vi "Begin.vi"(8 "error in":errorcluster) -> (0 "error out":errorcluster)   [LabVIEW 2016]
doc: "Called before other user functions, this VI is expected to open initial I/O refnums, load in file data, and do all program initialization. Notice that the <B>error out</B> terminal is simply used for data flow. Wiring it to other structures or subVIs ensures that this VI runs first."
uses:
  <vilib>/Rock Robotics/WPI/DriverStation/WPI_DriverStationRobotMode2.ctl
  <vilib>/Rock Robotics/WPI/Joystick/WPI_JoystickDeviceEnum.ctl
  <vilib>/Rock Robotics/SystemInterfaces/spilib/spi_bus.ctl
  <vilib>/Rock Robotics/WPI/SafetyOutput/WPI_SafetyOutputConfigMenu.ctl
  <vilib>/Rock Robotics/SystemInterfaces/DIO/FPGA_DIOPWMChannel.ctl
  <vilib>/Rock Robotics/WPI/Solenoid/WPI_SolenoidChannel.ctl
  <vilib>/Rock Robotics/SystemInterfaces/DIO/FPGA_DIOChannel.ctl
  <vilib>/Rock Robotics/WPI/Encoder/WPI_EncoderType.ctl
  <vilib>/Rock Robotics/SystemInterfaces/AI/FPGA_AIChannel.ctl
  Robot Global Data.vi
  navX Library v2/IO/Open/Z900_navX_Open_SPI.vi
  <vilib>/Rock Robotics/WPI/MotorControl/WPI_MotorControlOpen VictorSP.vi
  <vilib>/Rock Robotics/WPI/Solenoid/WPI_SolenoidOpenSingle.vi
  <vilib>/Rock Robotics/WPI/RobotDrive/WPI_RobotDriveOpen4MotorWithVictorSP.vi
  <vilib>/Rock Robotics/WPI/Counter/WPI_CounterDigitalInputToDigitalSource.vi
  <vilib>/Rock Robotics/WPI/Utilities/WPI_GetSetVariantRefNum.vi
  navX Library v2/navX Library v2.lvlib
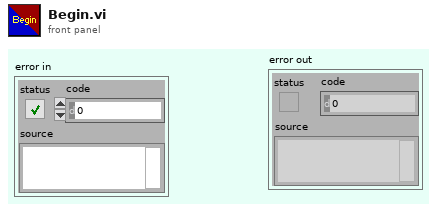
[diagram p1: front panel]
types:
  T1 = typedef "FPGA_AIChannel.ctl" = enum8{"AI 0", "AI 1", "AI 2", "AI 3", "AI MXP 0", "AI MXP 1", "AI MXP 2", "AI MXP 3", "Invalid"}
  T2 = typedef "WPI_EncoderType.ctl" = enum16{"1x", "2x", "4x"}
  T3 = typedef "FPGA_DIOChannel.ctl" = enum8{"DIO 0", "DIO 1", "DIO 2", "DIO 3", "DIO 4", "DIO 5", "DIO 6", "DIO 7", "DIO 8", "DIO 9", "DIO MXP 0", "DIO MXP 1", "DIO MXP 2", "DIO MXP 3", "DIO MXP 4", "DIO MXP 5", "DIO MXP 6", "DIO MXP 7", "DIO MXP 8", "DIO MXP 9", "DIO MXP 10", "DIO MXP 11", "DIO MXP 12", "DIO MXP 13", "DIO MXP 14", "DIO MXP 15", "SPI Port CS1", "SPI Port CS2", "SPI Port CS3", "SPI Port MISO", "SPI Port MOSI", "Invalid"}
  T4 = typedef "FPGA_DIOPWMChannel.ctl" = enum8{"PWM 0", "PWM 1", "PWM 2", "PWM 3", "PWM 4", "PWM 5", "PWM 6", "PWM 7", "PWM 8", "PWM 9", "PWM MXP 0", "PWM MXP 1", "PWM MXP 2", "PWM MXP 3", "PWM MXP 4", "PWM MXP 5", "PWM MXP 6", "PWM MXP 7", "PWM MXP 8", "PWM MXP 9", "Invalid"}
  T5 = typedef "WPI_SolenoidChannel.ctl" = enum8{"Solenoid 0", "Solenoid 1", "Solenoid 2", "Solenoid 3", "Solenoid 4", "Solenoid 5", "Solenoid 6", "Solenoid 7", "Invalid"}
  T6 = typedef "WPI_SafetyOutputConfigMenu.ctl" = enum16{"Enable", "Disable"}
  T7 = typedef "WPI_JoystickDeviceEnum.ctl" = enum16{"USB 0", "USB 1", "USB 2", "USB 3", "USB 4", "USB 5"}
  T8 = typedef "spi_bus.ctl" = enum16{"SPI On-Board, CS0", "SPI On-Board, CS1", "SPI On-Board, CS2", "SPI On-Board, CS3", "SPI MXP", "Invalid"}
  T9 = typedef "WPI_DriverStationRobotMode2.ctl" = enum16{"Autonomous Disabled", "Autonomous Enabled", "Teleop Disabled", "Teleop Enabled", "Disconnected", "Finish", "Test Disabled", "Test Enabled", "Emergency Stopped"}
  T10 = typedef "WPI_JoystickDevRef.ctl" = cluster{"Device":T7}
  T11 = typedef "WPI_MotorControlDeviceRef.ctl" = cluster{"DeviceStatus":errorcluster, "Type":T12, "PWM":cluster{"PWM Channel":T4, "DeadBand":T13}, "CAN":cluster{"Device Number":u8, "SetOutput VI Ref":variant, "GetOutput VI Ref":variant, "Enable VI Ref":variant, "Disable VI Ref":variant, "Data":variant}, "Invert":bool}
  T12 = typedef "WPI_MotorControlType.ctl" = enum16{"PWM", "CAN"}
  T13 = typedef "WPI_PWMDeadband.ctl" = cluster{"Name":string, "maxPositivePwm":i32, "minPositivePwm":i32, "centerPwm":i32, "maxNegativePwm":i32, "minNegativePwm":i32, "angularRange":u16}
  T14 = typedef "WPI_RobotDriveDevRef.ctl" = cluster{"DevStatus":errorcluster, "Motors[]":T11[], "Square Inputs":bool, "Max Output":dbl}
  T15 = typedef "WPI_CompressorDevRef.ctl" = cluster{"DevStatus":errorcluster, "Pneumatics Control Module":u8}
  T16 = typedef "WPI_SolenoidDevRef.ctl" = cluster{"DevStatus":errorcluster, "Pneumatics Control Module":u8, "Forward Solenoid Channel":T5, "Reverse Solenoid Channel":T5}
  T17 = typedef "WPI_DigitalInputDevRef.ctl" = cluster{"DevStatus":errorcluster, "DIO Channel":T3}
  T18 = typedef "navX Library v2.lvlib/Z900_navX_DeviceTypeDef.ctl" = cluster{"Interface":cluster{"Protocol":T19, "Update Rate (4Hz-100Hz)":u8, "navX Open TypeDef":variant}, "Notify Packet":refnum<notifier>, "Loop VI Refnum":refnum<vi>, "Ready to Close Occurrence Refnum":refnum<k4>}
  T19 = typedef "navX Library v2.lvlib/Z900_navX_ProtocolTypeDef.ctl" = enum16{"SERIAL", "I2C", "SPI"}
  T20 = typedef "WPI_AnalogChannelDevRef.ctl" = cluster{"DevStatus":errorcluster, "Analog Channel":T1}
  T21 = typedef "FPGA_CounterEncoderSourceConvertionLVSourceType.ctl" = cluster{"DevStatus":errorcluster, "AnalogTriggerMode?":bool, "DigitalMode":cluster{"DIO Channel":T22}, "AnalogTriggerMode":cluster{"AnalogTriggerIndex":T23, "OutputType":T24}}
  T22 = typedef "FPGA_DIODigitalSourceChannel.ctl" = enum8{"DIO 0", "DIO 1", "DIO 2", "DIO 3", "DIO 4", "DIO 5", "DIO 6", "DIO 7", "DIO 8", "DIO 9", "DIO MXP 0", "DIO MXP 1", "DIO MXP 2", "DIO MXP 3", "DIO MXP 4", "DIO MXP 5", "DIO MXP 6", "DIO MXP 7", "DIO MXP 8", "DIO MXP 9", "DIO MXP 10", "DIO MXP 11", "DIO MXP 12", "DIO MXP 13", "DIO MXP 14", "DIO MXP 15", "Disabled"}
  T23 = typedef "FPGA_AnalogTriggerIndex.ctl" = enum8{"Trig 0", "Trig 1", "Trig 2", "Trig 3", "Trig 4", "Trig 5", "Trig 6", "Trig 7", "Invalid"}
  T24 = typedef "FPGA_AnalogTriggerOutType.ctl" = enum16{"InWindow", "TriggerState", "Rising", "Falling"}
  T25 = typedef "WPI_EncoderDevRef.ctl" = cluster{"DevStatus":errorcluster, "EncoderIndex":T26, "CounterIndex":T27, "DistancePerCount":dbl, "Decoding Type":T2}
  T26 = typedef "FPGA_EncoderIdx.ctl" = enum8{"Enc 0", "Enc 1", "Enc 2", "Enc 3", "Enc 4", "Enc 5", "Enc 6", "Enc 7", "Invalid"}
  T27 = typedef "FPGA_CounterCtrSystemIndex.ctl" = enum8{"Ctr 0", "Ctr 1", "Ctr 2", "Ctr 3", "Ctr 4", "Ctr 5", "Ctr 6", "Ctr 7", "Invalid"}
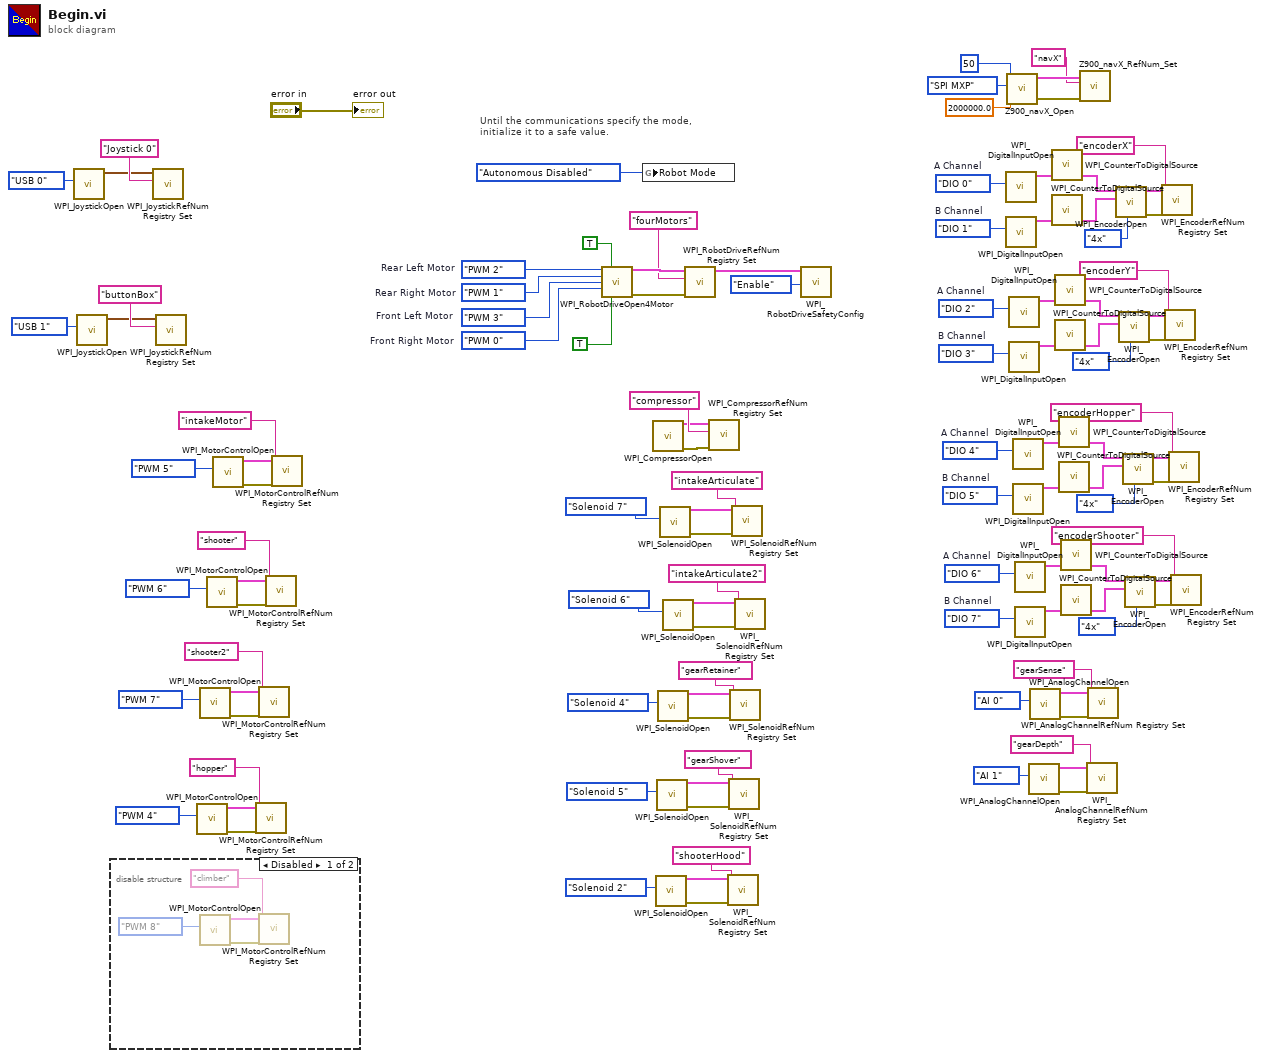
[diagram p0: block diagram]
diagram:
  w18 = FPGA_DIOChannel."DIO 7"  # B Channel
  w17 = FPGA_DIOChannel."DIO 6"  # A Channel
  w28 = FPGA_DIOChannel."DIO 5"  # B Channel
  w27 = FPGA_DIOChannel."DIO 4"  # A Channel
  w38 = FPGA_DIOChannel."DIO 3"  # B Channel
  w37 = FPGA_DIOChannel."DIO 2"  # A Channel
  w48 = FPGA_DIOChannel."DIO 1"  # B Channel
  w47 = FPGA_DIOChannel."DIO 0"  # A Channel
  w90 = FPGA_DIOPWMChannel."PWM 0"  # Front Right Motor
  w91 = FPGA_DIOPWMChannel."PWM 3"  # Front Left Motor
  w92 = FPGA_DIOPWMChannel."PWM 1"  # Rear Right Motor
  w93 = FPGA_DIOPWMChannel."PWM 2"  # Rear Left Motor
  # "Until the communications specify the mode,\ninitialize it to a safe value."
  n1 = call <vilib>:"WPI_JoystickOpen.vi"("JoystickDevice"=WPI_JoystickDeviceEnum."USB 0") -> ("JoystickDevRef"=w110:T10)  [unwired: 10 in]
  n2 = call <vilib>:"WPI_JoystickOpen.vi"("JoystickDevice"=WPI_JoystickDeviceEnum."USB 1") -> ("JoystickDevRef"=w100:T10)  [unwired: 10 in]
  n3 = disable-structure shown="Disabled" {
    frame Disabled {
      n4 = call-poly <vilib>:"WPI_MotorControlOpen.vi"("PWM Channel"=FPGA_DIOPWMChannel."PWM 8") -> ("error out"=w113:errorcluster, "MotorControlDeviceRef"=w114:T11)  [unwired: 9 in]
      n5 = call <vilib>:"WPI_MotorControlRefNum Registry Set.vi"("error in (no error)"=w113, "refnum name"="climber", "MotorControlDevRef"=w114) -> ()  [unwired: 7 in, 2 out]
    }
    frame Enabled {
    }
  }
  n6 = call <vilib>:"WPI_JoystickRefNum Registry Set.vi"("refnum name"="Joystick 0", "JoystickDevRef"=w110) -> ()  [unwired: 8 in, 2 out]
  n7 = call <vilib>:"WPI_JoystickRefNum Registry Set.vi"("refnum name"="buttonBox", "JoystickDevRef"=w100) -> ()  [unwired: 8 in, 2 out]
  n8 = call-poly <vilib>:"WPI_MotorControlOpen.vi"("PWM Channel"=FPGA_DIOPWMChannel."PWM 4") -> ("error out"=w55:errorcluster, "MotorControlDeviceRef"=w56:T11)  [unwired: 9 in]
  n9 = call-poly <vilib>:"WPI_MotorControlOpen.vi"("PWM Channel"=FPGA_DIOPWMChannel."PWM 7") -> ("error out"=w51:errorcluster, "MotorControlDeviceRef"=w52:T11)  [unwired: 9 in]
  n10 = call-poly <vilib>:"WPI_MotorControlOpen.vi"("PWM Channel"=FPGA_DIOPWMChannel."PWM 6") -> ("error out"=w59:errorcluster, "MotorControlDeviceRef"=w60:T11)  [unwired: 9 in]
  n11 = call-poly <vilib>:"WPI_MotorControlOpen.vi"("PWM Channel"=FPGA_DIOPWMChannel."PWM 5") -> ("error out"=w86:errorcluster, "MotorControlDeviceRef"=w87:T11)  [unwired: 9 in]
  n12 = call <vilib>:"WPI_MotorControlRefNum Registry Set.vi"("error in (no error)"=w55, "refnum name"="hopper", "MotorControlDevRef"=w56) -> ()  [unwired: 7 in, 2 out]
  n13 = call <vilib>:"WPI_MotorControlRefNum Registry Set.vi"("error in (no error)"=w51, "refnum name"="shooter2", "MotorControlDevRef"=w52) -> ()  [unwired: 7 in, 2 out]
  n14 = call <vilib>:"WPI_MotorControlRefNum Registry Set.vi"("error in (no error)"=w59, "refnum name"="shooter", "MotorControlDevRef"=w60) -> ()  [unwired: 7 in, 2 out]
  n15 = call <vilib>:"WPI_MotorControlRefNum Registry Set.vi"("error in (no error)"=w86, "refnum name"="intakeMotor", "MotorControlDevRef"=w87) -> ()  [unwired: 7 in, 2 out]
  n16 = call-poly <vilib>:"WPI_RobotDriveOpen4Motor.vi"("Rear Left Motor"=w93, "Rear Left Motor Inverted"=TRUE ("Rear Right Motor Inverted"), "Rear Right Motor"=w92, "Front Left Motor"=w91, "Front Right Motor"=w90, "Front Left Motor Inverted"=TRUE ("Front Right Motor Inverted")) -> ("RobotDriveDevRef"=w98:T14, "error out"=w96:errorcluster)  [unwired: 8 in]
  n17 = global write "Robot Global Data.vi" "Robot Mode"(WPI_DriverStationRobotMode2."Autonomous Disabled" ("Robot Mode")) -> ()
  n18 = call <vilib>:"WPI_CompressorOpen.vi"() -> ("CompressorDevRef"=w76:T15, "error out"=w75:errorcluster)  [unwired: 14 in]
  n19 = call-poly <vilib>:"WPI_SolenoidOpen.vi"("Solenoid Channel"=WPI_SolenoidChannel."Solenoid 2") -> ("error out"=w64:errorcluster, "SolenoidDevRef"=w63:T16)  [unwired: 9 in]
  n20 = call-poly <vilib>:"WPI_SolenoidOpen.vi"("Solenoid Channel"=WPI_SolenoidChannel."Solenoid 5") -> ("error out"=w68:errorcluster, "SolenoidDevRef"=w67:T16)  [unwired: 9 in]
  n21 = call-poly <vilib>:"WPI_SolenoidOpen.vi"("Solenoid Channel"=WPI_SolenoidChannel."Solenoid 4") -> ("error out"=w82:errorcluster, "SolenoidDevRef"=w81:T16)  [unwired: 9 in]
  n22 = call-poly <vilib>:"WPI_SolenoidOpen.vi"("Solenoid Channel"=WPI_SolenoidChannel."Solenoid 7") -> ("error out"=w79:errorcluster, "SolenoidDevRef"=w78:T16)  [unwired: 9 in]
  n23 = call-poly <vilib>:"WPI_SolenoidOpen.vi"("Solenoid Channel"=WPI_SolenoidChannel."Solenoid 6") -> ("error out"=w72:errorcluster, "SolenoidDevRef"=w71:T16)  [unwired: 9 in]
  n24 = call <vilib>:"WPI_RobotDriveRefNum Registry Set.vi"("error in (no error)"=w96, "refnum name"="fourMotors", "RobotDriveDevRef"=w98) -> ("RobotDriveDevRef"=w95:T14)  [unwired: 1 in, 7 out]
  n25 = call <vilib>:"WPI_CompressorRefNum Registry Set.vi"("error in (no error)"=w75, "refnum name"="compressor", "CompressorDevRef"=w76) -> ()  [unwired: 7 in, 2 out]
  n26 = call <vilib>:"WPI_SolenoidRefNum Registry Set.vi"("error in (no error)"=w64, "refnum name"="shooterHood", "SolenoidDevRef"=w63) -> ()  [unwired: 7 in, 2 out]
  n27 = call <vilib>:"WPI_SolenoidRefNum Registry Set.vi"("error in (no error)"=w68, "refnum name"="gearShover", "SolenoidDevRef"=w67) -> ()  [unwired: 7 in, 2 out]
  n28 = call <vilib>:"WPI_SolenoidRefNum Registry Set.vi"("error in (no error)"=w82, "refnum name"="gearRetainer", "SolenoidDevRef"=w81) -> ()  [unwired: 7 in, 2 out]
  n29 = call <vilib>:"WPI_SolenoidRefNum Registry Set.vi"("error in (no error)"=w79, "refnum name"="intakeArticulate", "SolenoidDevRef"=w78) -> ()  [unwired: 7 in, 2 out]
  n30 = call <vilib>:"WPI_SolenoidRefNum Registry Set.vi"("error in (no error)"=w72, "refnum name"="intakeArticulate2", "SolenoidDevRef"=w71) -> ()  [unwired: 7 in, 2 out]
  n31 = call <vilib>:"WPI_RobotDriveSafetyConfig.vi"("mode"=WPI_SafetyOutputConfigMenu."Enable", "RobotDriveDevRef"=w95) -> ()  [unwired: 8 in, 2 out]
  n32 = call <vilib>:"WPI_DigitalInputOpen.vi"("DIO Channel"=w47) -> ("DigitalInputDevRef"=w44:T17)  [unwired: 1 in, 9 out]
  n33 = call <vilib>:"WPI_DigitalInputOpen.vi"("DIO Channel"=w48) -> ("DigitalInputDevRef"=w45:T17)  [unwired: 1 in, 9 out]
  n34 = call-poly "Z900_navX_Open.vi"("Clock Rate (Hz)"=2000000.0, "SPI Bus"=spi_bus."SPI MXP", "Update Rate (4Hz-60Hz)"=u8 50) -> ("error out"=w106:errorcluster, "navX Device"=w107:T18)  [unwired: 7 in]
  n35 = call <vilib>:"WPI_DigitalInputOpen.vi"("DIO Channel"=w37) -> ("DigitalInputDevRef"=w34:T17)  [unwired: 1 in, 9 out]
  n36 = call <vilib>:"WPI_DigitalInputOpen.vi"("DIO Channel"=w38) -> ("DigitalInputDevRef"=w35:T17)  [unwired: 1 in, 9 out]
  n37 = call <vilib>:"WPI_DigitalInputOpen.vi"("DIO Channel"=w27) -> ("DigitalInputDevRef"=w24:T17)  [unwired: 1 in, 9 out]
  n38 = call <vilib>:"WPI_DigitalInputOpen.vi"("DIO Channel"=w28) -> ("DigitalInputDevRef"=w25:T17)  [unwired: 1 in, 9 out]
  n39 = call <vilib>:"WPI_DigitalInputOpen.vi"("DIO Channel"=w17) -> ("DigitalInputDevRef"=w14:T17)  [unwired: 1 in, 9 out]
  n40 = call <vilib>:"WPI_DigitalInputOpen.vi"("DIO Channel"=w18) -> ("DigitalInputDevRef"=w15:T17)  [unwired: 1 in, 9 out]
  n41 = call <vilib>:"WPI_AnalogChannelOpen.vi"("Analog Channel"=FPGA_AIChannel."AI 1") -> ("error out"=w4:errorcluster, "AIDeviceRef"=w3:T20)  [unwired: 9 in]
  n42 = call <vilib>:"WPI_AnalogChannelOpen.vi"("Analog Channel"=FPGA_AIChannel."AI 0") -> ("error out"=w8:errorcluster, "AIDeviceRef"=w7:T20)  [unwired: 9 in]
  n43 = call-poly <vilib>:"WPI_CounterToDigitalSource.vi"("DigitalInputDevRef"=w44) -> ("Digital Source"=w43:T21)  [unwired: 6 out]
  n44 = call-poly <vilib>:"WPI_CounterToDigitalSource.vi"("DigitalInputDevRef"=w45) -> ("Digital Source"=w46:T21)  [unwired: 6 out]
  n45 = call-poly <vilib>:"WPI_CounterToDigitalSource.vi"("DigitalInputDevRef"=w34) -> ("Digital Source"=w33:T21)  [unwired: 6 out]
  n46 = call-poly <vilib>:"WPI_CounterToDigitalSource.vi"("DigitalInputDevRef"=w35) -> ("Digital Source"=w36:T21)  [unwired: 6 out]
  n47 = call-poly <vilib>:"WPI_CounterToDigitalSource.vi"("DigitalInputDevRef"=w24) -> ("Digital Source"=w23:T21)  [unwired: 6 out]
  n48 = call-poly <vilib>:"WPI_CounterToDigitalSource.vi"("DigitalInputDevRef"=w25) -> ("Digital Source"=w26:T21)  [unwired: 6 out]
  n49 = call-poly <vilib>:"WPI_CounterToDigitalSource.vi"("DigitalInputDevRef"=w14) -> ("Digital Source"=w13:T21)  [unwired: 6 out]
  n50 = call-poly <vilib>:"WPI_CounterToDigitalSource.vi"("DigitalInputDevRef"=w15) -> ("Digital Source"=w16:T21)  [unwired: 6 out]
  n51 = call "Z900_navX_RefNum_Set.vi"("error in (no error)"=w106, "refnum name"="navX", "navX Device"=w107) -> ()  [unwired: 7 in, 2 out]
  n52 = call <vilib>:"WPI_AnalogChannelRefNum Registry Set.vi"("error in (no error)"=w4, "refnum name"="gearDepth", "AIDeviceRef"=w3) -> ()  [unwired: 7 in, 2 out]
  n53 = call <vilib>:"WPI_AnalogChannelRefNum Registry Set.vi"("error in (no error)"=w8, "refnum name"="gearSense", "AIDeviceRef"=w7) -> ()  [unwired: 7 in, 2 out]
  n54 = call <vilib>:"WPI_EncoderOpen.vi"("Decoding Type"=WPI_EncoderType."4x", "BSource"=w46, "ASource"=w43) -> ("error out"=w42:errorcluster, "EncoderDevRef"=w41:T25)  [unwired: 5 in, 2 out]
  n55 = call <vilib>:"WPI_EncoderOpen.vi"("Decoding Type"=WPI_EncoderType."4x", "BSource"=w36, "ASource"=w33) -> ("error out"=w32:errorcluster, "EncoderDevRef"=w31:T25)  [unwired: 5 in, 2 out]
  n56 = call <vilib>:"WPI_EncoderOpen.vi"("Decoding Type"=WPI_EncoderType."4x", "BSource"=w26, "ASource"=w23) -> ("error out"=w22:errorcluster, "EncoderDevRef"=w21:T25)  [unwired: 5 in, 2 out]
  n57 = call <vilib>:"WPI_EncoderOpen.vi"("Decoding Type"=WPI_EncoderType."4x", "BSource"=w16, "ASource"=w13) -> ("error out"=w12:errorcluster, "EncoderDevRef"=w11:T25)  [unwired: 5 in, 2 out]
  n58 = call <vilib>:"WPI_EncoderRefNum Registry Set.vi"("error in (no error)"=w42, "refnum name"="encoderX", "EncoderDevRef"=w41) -> ()  [unwired: 7 in, 2 out]
  n59 = call <vilib>:"WPI_EncoderRefNum Registry Set.vi"("error in (no error)"=w32, "refnum name"="encoderY", "EncoderDevRef"=w31) -> ()  [unwired: 7 in, 2 out]
  n60 = call <vilib>:"WPI_EncoderRefNum Registry Set.vi"("error in (no error)"=w22, "refnum name"="encoderHopper", "EncoderDevRef"=w21) -> ()  [unwired: 7 in, 2 out]
  n61 = call <vilib>:"WPI_EncoderRefNum Registry Set.vi"("error in (no error)"=w12, "refnum name"="encoderShooter", "EncoderDevRef"=w11) -> ()  [unwired: 7 in, 2 out]
  "error out" <- "error in"
